vi "piezo2WriteClose.vi"   [LabVIEW 2017]
uses:
  globalDevices.vi
  <vilib>/DAQmx/write.llb/DAQmx Write (Analog DBL 1Chan 1Samp).vi
  <vilib>/DAQmx/create/channels.llb/DAQmx Create Channel (AO-Voltage-Basic).vi
  <vilib>/DAQmx/create/channels.llb/DAQmx Create Channel (AI-Voltage-Basic).vi
  <vilib>/DAQmx/read.llb/DAQmx Read (Analog DBL 1Chan 1Samp).vi
  Piezo/lvlib/Madlib.lvlib
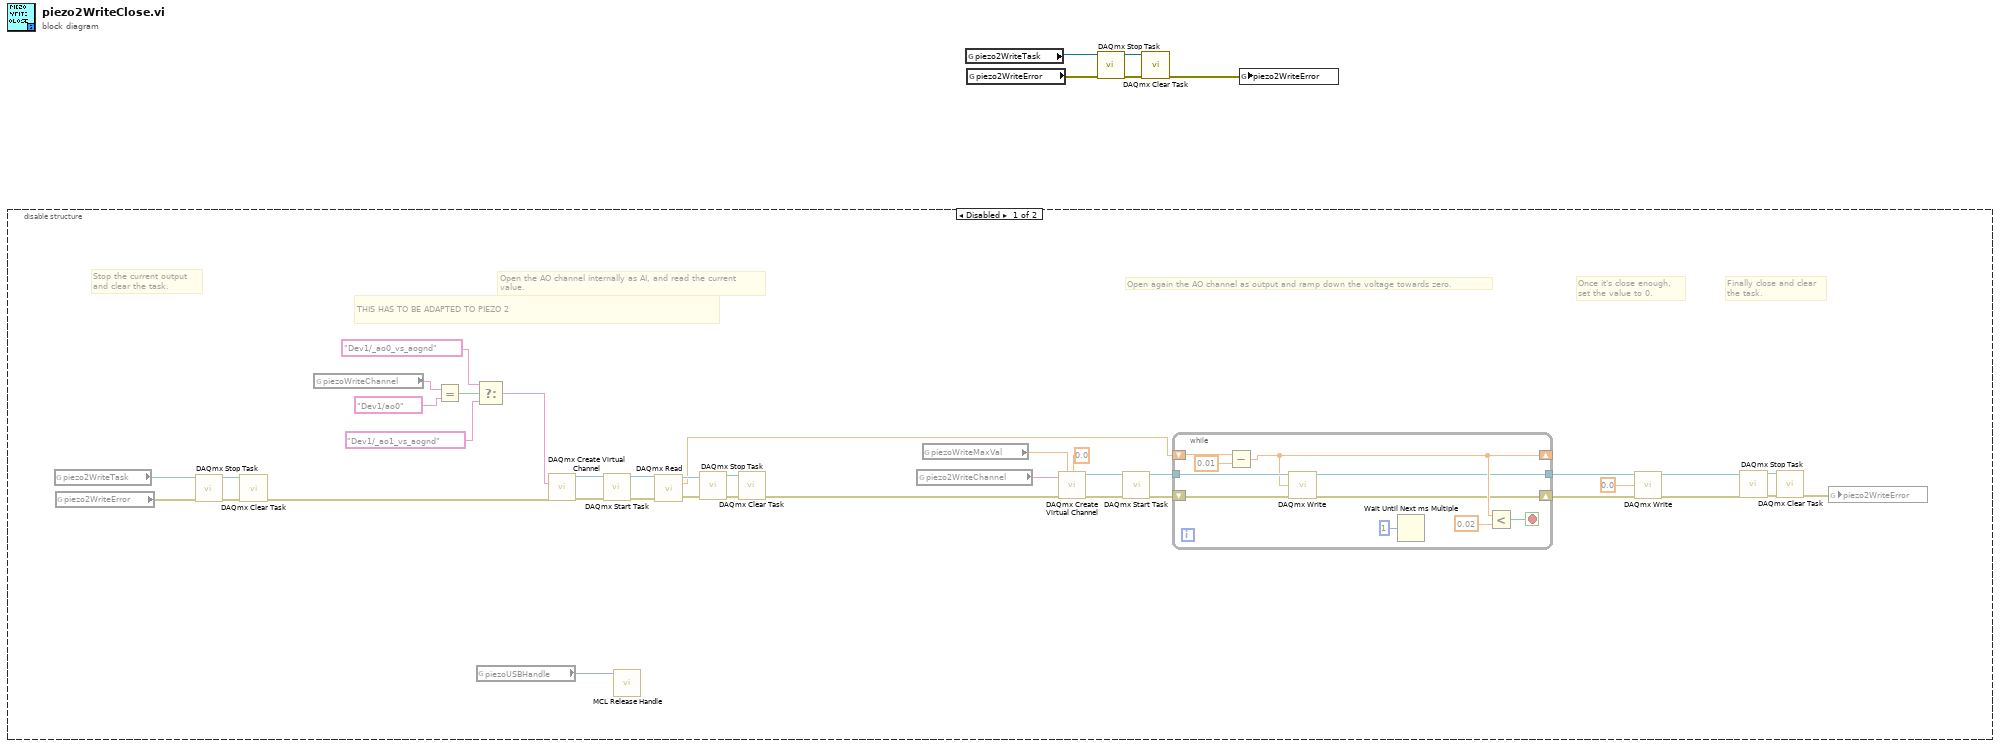
[diagram p0: block diagram]
diagram:
  n1 = disable-structure shown="Disabled" {
    frame Disabled {
      # "THIS HAS TO BE ADAPTED TO PIEZO 2"
      # "Finally close and clear\nthe task."
      # "Once it's close enough,\nset the value to 0."
      # "Open again the AO channel as output and ramp down the voltage towards zero."
      # "Open the AO channel internally as AI, and read the current\nvalue."
      # "Stop the current output\nand clear the task."
      n2 = global read "globalDevices.vi" "piezo2WriteTask"() -> (w41:refnum<k21>)
      n3 = global read "globalDevices.vi" "piezo2WriteError"() -> (w42:errorcluster)
      n4 = call <vilib>:"DAQmx Stop Task.vi"("task/channels in"=w41, "error in"=w42) -> ("task out"=w39:refnum<k21>, "error out"=w40:errorcluster)  [unwired: 12 in]
      n5 = call <vilib>:"DAQmx Clear Task.vi"("task in"=w39, "error in"=w40) -> ("error out"=w18:errorcluster)  [unwired: 13 in]
      n6 = global read "globalDevices.vi" "piezoWriteChannel"() -> (w24:tag)
      n7 = Equal?(x=w24, y=tag "Dev1/ao0" ("physical channels")) -> (x = y?=w22:bool)
      n8 = global read "globalDevices.vi" "piezoUSBHandle"() -> (w6:i32)
      n9 = Select(t=tag "Dev1/_ao0_vs_aognd" ("physical channels"), s=w22, f=tag "Dev1/_ao1_vs_aognd" ("physical channels")) -> (s? t:f=w19:tag)
      n10 = call-poly <vilib>:"DAQmx Create Virtual Channel.vi"("physical channels"=w19, "error in"=w18) -> ("task out"=w30:refnum<k21>, "error out"=w17:errorcluster)  [unwired: 12 in]
      n11 = call <vilib>:"DAQmx Start Task.vi"("task/channels in"=w30, "error in"=w17) -> ("task out"=w29:refnum<k21>, "error out"=w16:errorcluster)  [unwired: 12 in]
      n12 = call "MCL Release Handle.vi"("handle"=w6) -> ()  [unwired: 11 in]
      n13 = call-poly <vilib>:"DAQmx Read.vi"("task/channels in"=w29, "error in"=w16) -> ("task out"=w28:refnum<k21>, "data"=w26:dbl, "error out"=w15:errorcluster)  [unwired: 11 in]
      n14 = call <vilib>:"DAQmx Stop Task.vi"("task/channels in"=w28, "error in"=w15) -> ("task out"=w32:refnum<k21>, "error out"=w31:errorcluster)  [unwired: 12 in]
      n15 = call <vilib>:"DAQmx Clear Task.vi"("task in"=w32, "error in"=w31) -> ("error out"=w27:errorcluster)  [unwired: 13 in]
      n16 = global read "globalDevices.vi" "piezo2WriteChannel"() -> (w25:tag)
      n17 = global read "globalDevices.vi" "piezoWriteMaxVal"() -> (w33:dbl)
      n18 = call-poly <vilib>:"DAQmx Create Virtual Channel.vi"("maximum value"=w33, "minimum value"=0.0, "physical channels"=w25, "error in"=w27) -> ("task out"=w35:refnum<k21>, "error out"=w14:errorcluster)  [unwired: 10 in]
      n19 = call <vilib>:"DAQmx Start Task.vi"("task/channels in"=w35, "error in"=w14) -> ("task out"=w34:refnum<k21>, "error out"=w13:errorcluster)  [unwired: 12 in]
      n20 = while {
        shift-right: [w47] -> _
        shift-left: w26 -> [w52]
        tunnel: w34 -> [w48]
        tunnel: [w46] -> w12
        shift-right: [w43] -> w11
        shift-left: w13 -> [w44]
        stop <- w49 stop-if-true
        n21 = Subtract(x=w52, y=0.01) -> (x-y=w47:dbl)
        n22 = call-poly <vilib>:"DAQmx Write.vi"("task/channels in"=w48, "data"=w47, "error in"=w44) -> ("task out"=w46:refnum<k21>, "error out"=w43:errorcluster)  [unwired: 10 in, 1 out]
        n23 = Wait Until Next ms Multiple(millisecond multiple=u32 1) -> ()  [unwired: 1 out]
        n24 = Less?(x=w47, y=0.02) -> (x < y?=w49:bool)
      }
      n25 = call-poly <vilib>:"DAQmx Write.vi"("task/channels in"=w12, "data"=0.0, "error in"=w11) -> ("task out"=w10:refnum<k21>, "error out"=w9:errorcluster)  [unwired: 10 in, 1 out]
      n26 = call <vilib>:"DAQmx Stop Task.vi"("task/channels in"=w10, "error in"=w9) -> ("task out"=w38:refnum<k21>, "error out"=w37:errorcluster)  [unwired: 12 in]
      n27 = call <vilib>:"DAQmx Clear Task.vi"("task in"=w38, "error in"=w37) -> ("error out"=w7:errorcluster)  [unwired: 13 in]
      n28 = global write "globalDevices.vi" "piezo2WriteError"(w7) -> ()
    }
    frame Enabled {
    }
  }
  n29 = global read "globalDevices.vi" "piezo2WriteTask"() -> (w3:refnum<k21>)
  n30 = global read "globalDevices.vi" "piezo2WriteError"() -> (w1:errorcluster)
  n31 = call <vilib>:"DAQmx Stop Task.vi"("task/channels in"=w3, "error in"=w1) -> ("task out"=w4:refnum<k21>, "error out"=w5:errorcluster)  [unwired: 12 in]
  n32 = call <vilib>:"DAQmx Clear Task.vi"("task in"=w4, "error in"=w5) -> ("error out"=w2:errorcluster)  [unwired: 13 in]
  n33 = global write "globalDevices.vi" "piezo2WriteError"(w2) -> ()
